vi "MagnetometerStateMachineV1.vi"() -> ()   [LabVIEW 2014]
uses:
  <vilib>/MakerHub/LINX/Private/Local IO/LinxI2cWrite.vi
  <vilib>/MakerHub/LINX/Public/Utilities/Check Channel.vi
  <vilib>/MakerHub/LINX/Public/Utilities/Open Serial.vi
  <vilib>/MakerHub/LINX/Private/Utilties/Generate Error.vi
  <instrlib>/Stanford Research 830/Public/Data/Read (All Parameters).vi
  <vilib>/MakerHub/LINX/LMH-LINX.lvlib
  <instrlib>/Stanford Research 830/Stanford Research 830.lvlib
panel:
  out "SRS-T":dbl
  out "SRS-R":dbl
  out "SRS-Y":dbl
  out "Parameter Values":T1
  out "XY Graph":T2(graph)
  out "SRS-X":dbl
  in  "Time Constant (8: 100ms)":u16(ring)=8 items=["10 us", "30 us", "100 us", "300 us", "1 ms", "3 ms", "10 ms", "30 ms", "100 ms", "300 ms", "1 s", "3 s", "10 s", "30 s", "100 s", "300 s", "1 ks", "3 ks", "10 ks", "30 ks"]
  in  "Internal Reference Frequency (1000 Hz)":dbl=1000.0
  in  "Sine Output Amplitude (1 V)":dbl=1.0
  in  "Sensitivity (26: 1 V/uA)":i16(ring)=26 items=["Auto Gain"=-1, "2 nV/fA"=0, "5 nV/fA"=1, "10 nV/fA"=2, "20 nV/fA"=3, "50 nV/fA"=4, "100 nV/fA"=5, "200 nV/fA"=6, "500 nV/fA"=7, "1 uV/pA"=8, "2 uV/pA"=9, "5 uV/pA"=10, "10 uV/pA"=11, "20 uV/pA"=12, "50 uV/pA"=13, "100 uV/pA"=14, "200 uV/pA"=15, "500 uV/pA"=16, "1 mV/nA"=17, "2 mV/nA"=18, "5 mV/nA"=19, "10 mV/nA"=20, "20 mV/nA"=21, "50 mV/nA"=22, "100 mV/nA"=23, "200 mV/nA"=24, "500 mV/mA"=25, "1 V/uA"=26]
  in  "Dynamic Reserve (2: Low Noise)":i16(ring)=2 items=["High Reserve"=0, "Normal"=1, "Low Noise"=2, "Auto Reserve"=-1]
  in  "Reference Source (1: Internal)":u16(ring)=1 items=["External", "Internal"]
  in  "Input Coupling (0: AC)":u16(ring) items=["AC", "DC"]
  in  "Input Connection (0: Single-Ended Voltage)":u16(ring) items=["Single-Ended Voltage", "Differential Voltage", "1 MOhm Current Gain", "100 MOhm Current Gain"]
  in  "Current DAC Value":dbl
  in  "Max H Field (Oe)":sgl min=0 max=900 step=0.1
  in  "DAC Zeroing Voltage":dbl=2.5 min=0.0 max=5.0 step=0.001 format="%#_6f"
  out "Magnetic Field (Oe)":dbl
  in  "Choices":T3(ring)
  in  "End It All!":bool
  out "Error Out":errorcluster={"status"=FALSE, "code"=1073676294, "source"="VISA Read in LVH-LINX.lvlib:Device.lvlib:Serial Read.vi->LVH-LINX.lvlib:Device.lvlib:Wait For Packet.vi->LVH-LINX.lvlib:Device.lvlib:Send Command.vi->LVH-LINX.lvlib:Device.lvlib:Get DIO Channels.vi->LVH-LINX.lvlib:Device.lvlib:Load Device Config.vi->LVH-LINX.lvlib:Device.lvlib:Initialize Device.vi->LVH-LINX.lvlib:Initialize.vi->Untitled 2"}
  out "Device Name":string
  in  "Arduino Port":refnum<visa-resource-name>="N/A"
  # "Enter the voltage to get\nthe magnetic field to be zero."
  # "Input Signal"
  # "Reference"
  # "Sensitivity and Reserve"
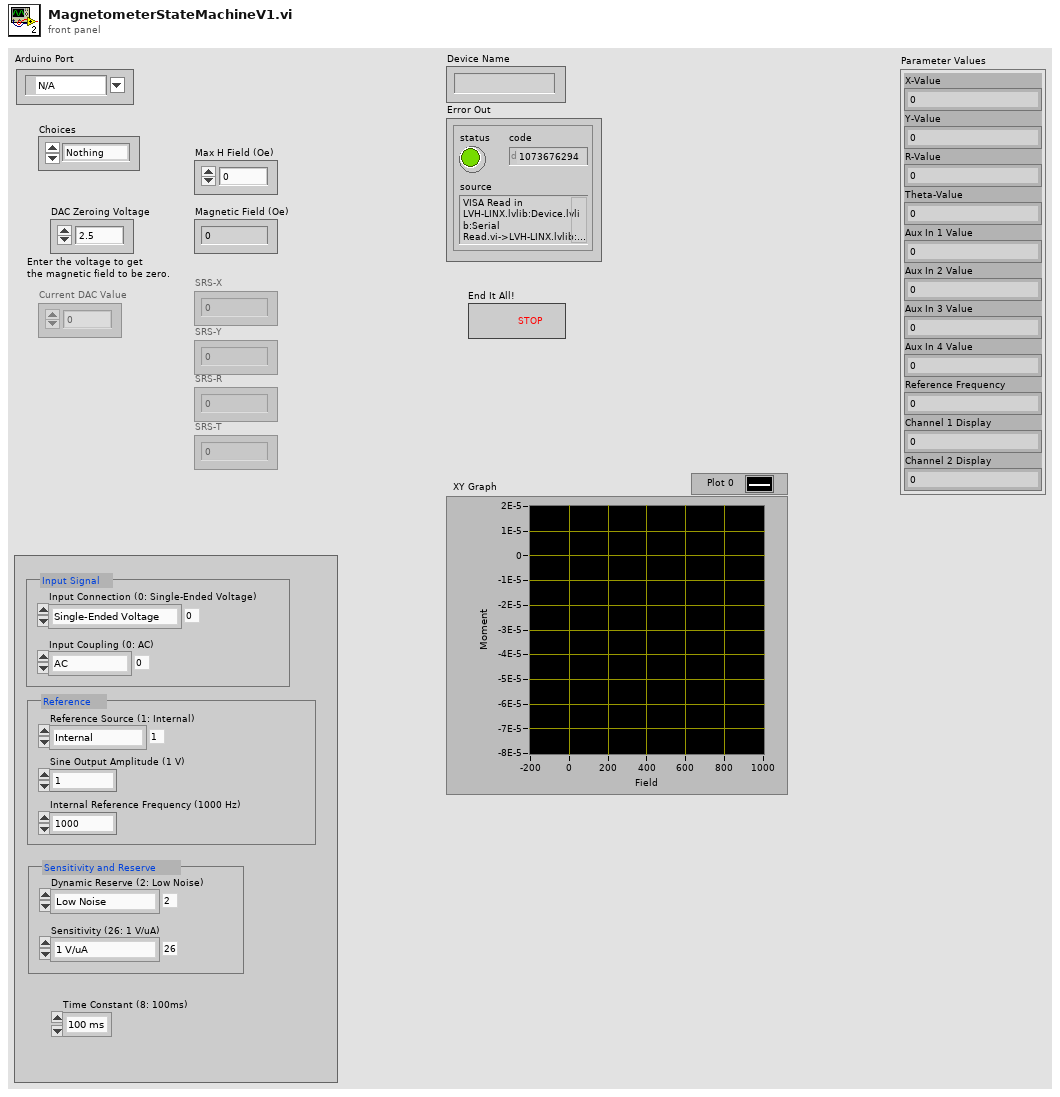
[diagram p1: front panel]
types:
  T1 = cluster{"X-Value":dbl, "Y-Value":dbl, "R-Value":dbl, "Theta-Value":dbl, "Aux In 1 Value":dbl, "Aux In 2 Value":dbl, "Aux In 3 Value":dbl, "Aux In 4 Value":dbl, "Reference Frequency":dbl, "Channel 1 Display":dbl, "Channel 2 Display":dbl}
  T2 = cluster{"Magnetic Field (Oe)":dbl, "Moment":dbl}[]
  T3 = enum16{"Nothing", "Hysteresis", "MvsT", "SetTemperature", "ZeroHField"}
  T4 = typedef "LMH-LINX.lvlib/LINX Ref.ctl" = cluster{"IO":T5, "Interface":T6, "LINX Device Config":T7}
  T5 = typedef "LMH-LINX.lvlib/Platform.ctl" = enum16{"Remote", "Local"}
  T6 = typedef "LMH-LINX.lvlib/Interface.ctl" = enum16{"Serial", "TCP"}
  T7 = typedef "LMH-LINX.lvlib/Device.lvlib/LINX Device Config.ctl" = cluster{"Interface":T6, "COM Port":refnum<visa-resource-name>, "TCP Configuration":T8, "Device Family":u8, "Device ID":u8, "Device Name":string, "TCP Ref":refnum<k5>, "Channels":T9}
  T8 = typedef "LMH-LINX.lvlib/Device.lvlib/TCP Config.ctl" = cluster{"IP Address":string, "Port":u16}
  T9 = typedef "LMH-LINX.lvlib/Channels.ctl" = cluster{"DI":u8[], "DO":u8[], "AI":u8[], "AO":u8[], "PWM":u8[], "QE":u8[], "UART":u8[], "I2C 2":u8[], "SPI":u8[], "CAN":u8[], "Servo":u8[], "AI Ref (V)":dbl, "AI Resolution (Bits)":u8, "AO Ref (V)":dbl, "AO Resolution (Bits)":u8}
  T10 = cluster{"Magnetic Field (Oe)":dbl, "SRS-X":dbl}[]
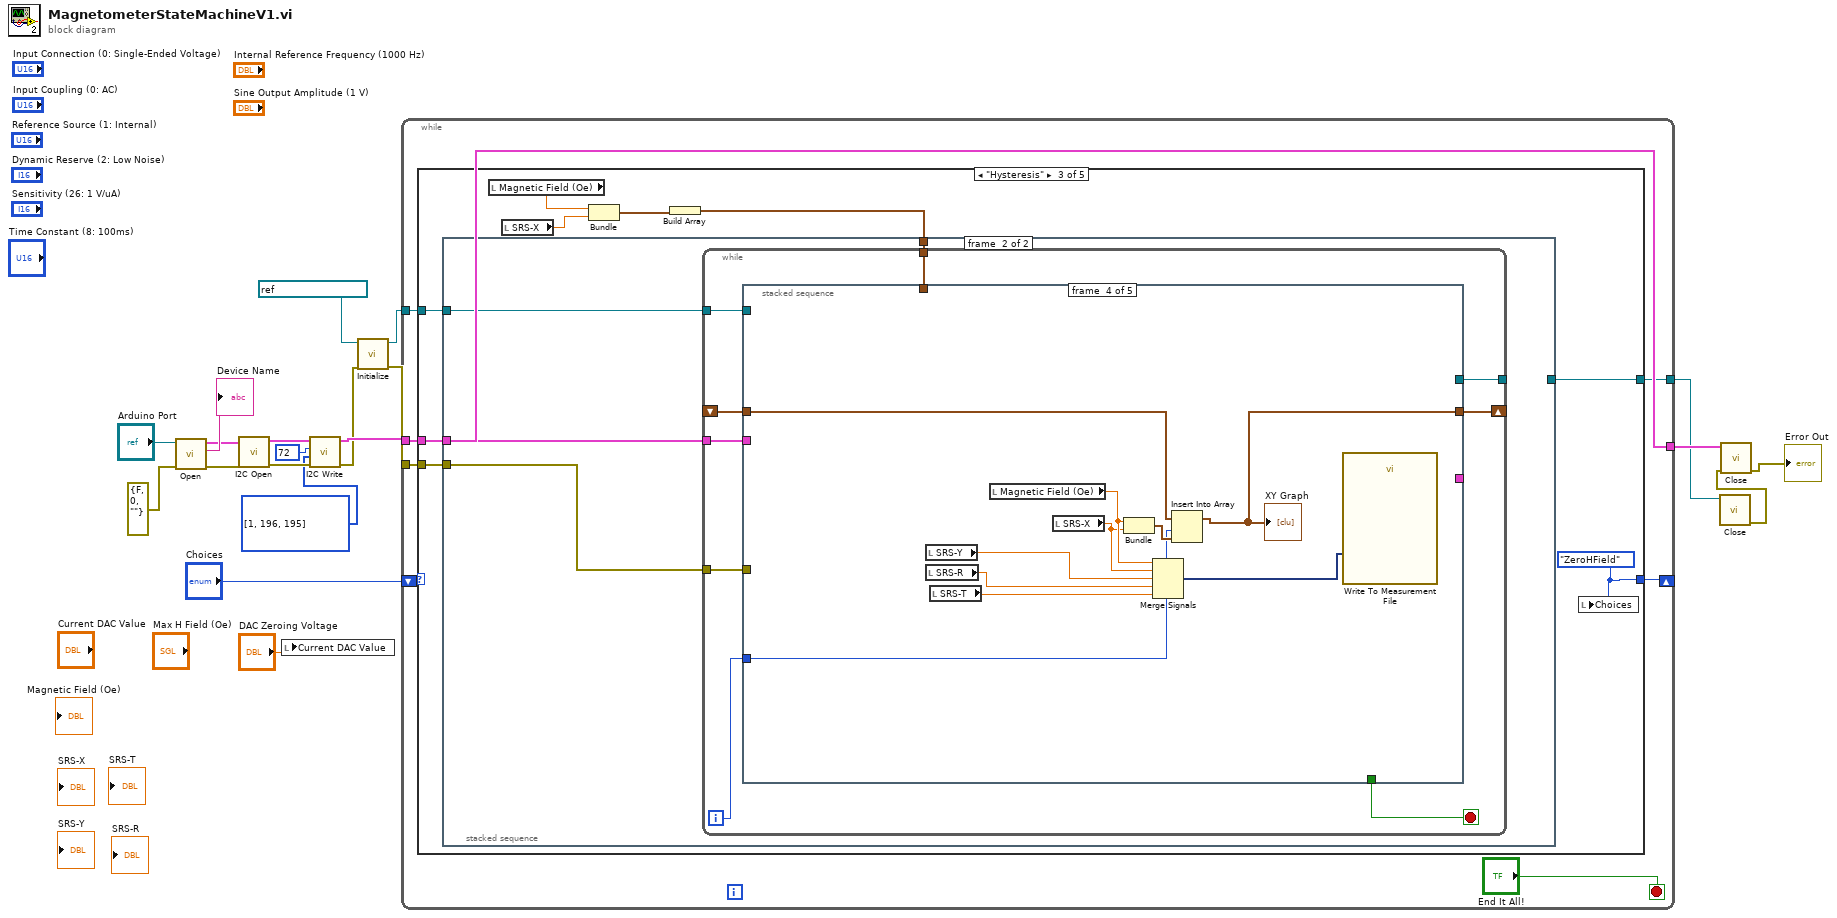
[diagram p0: block diagram]
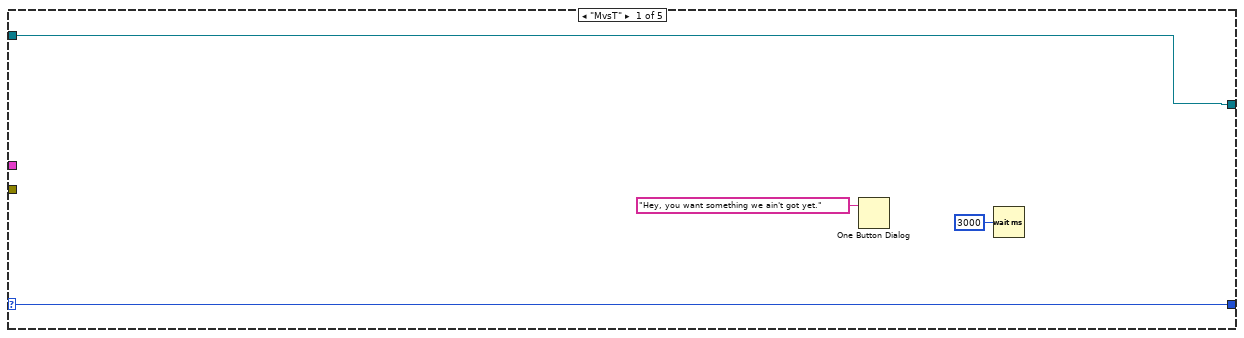
[diagram p2: hidden frame]
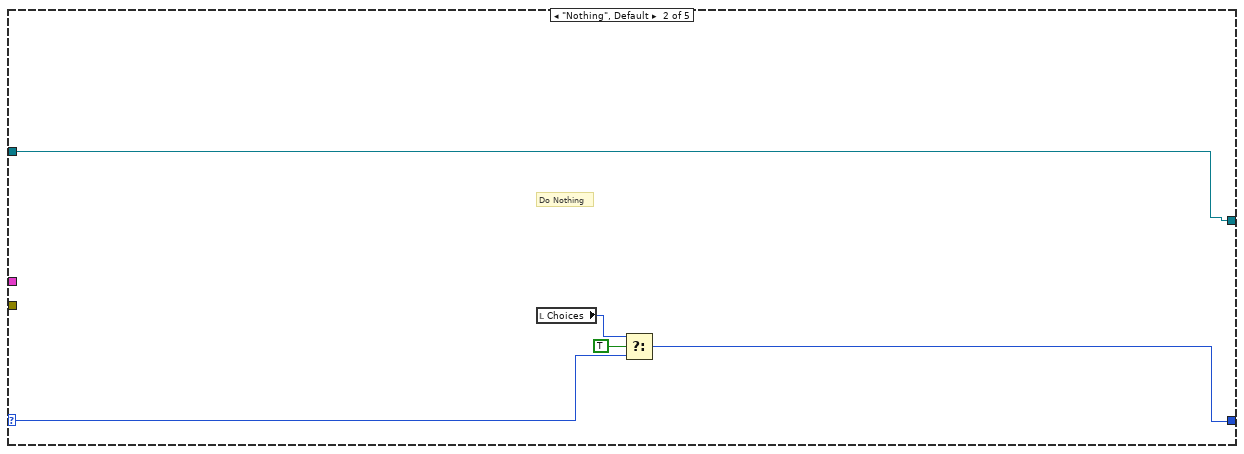
[diagram p3: hidden frame]
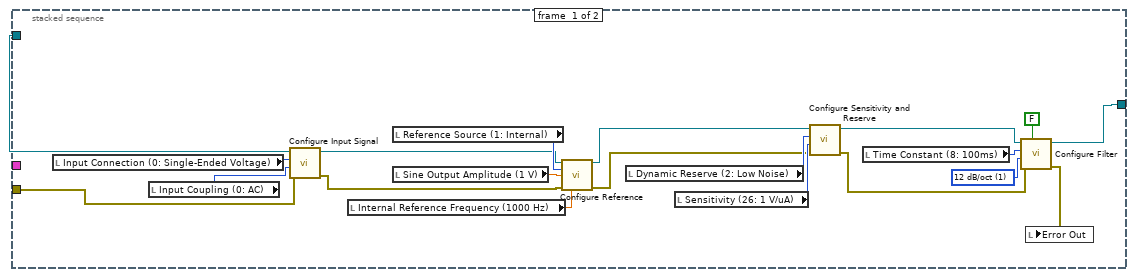
[diagram p4: hidden frame]
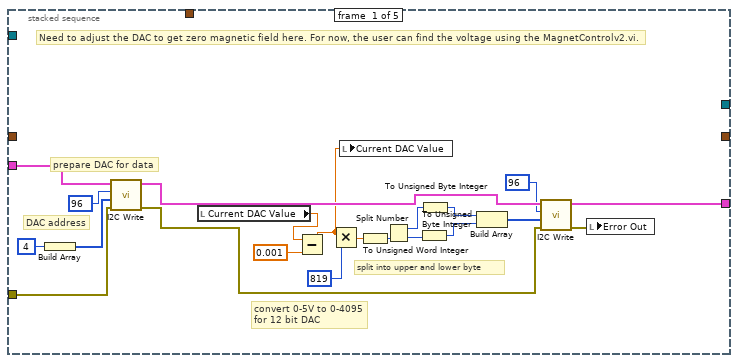
[diagram p5: hidden frame]
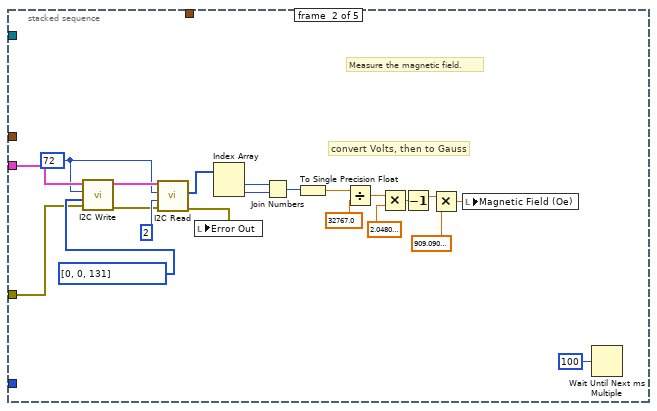
[diagram p6: hidden frame]
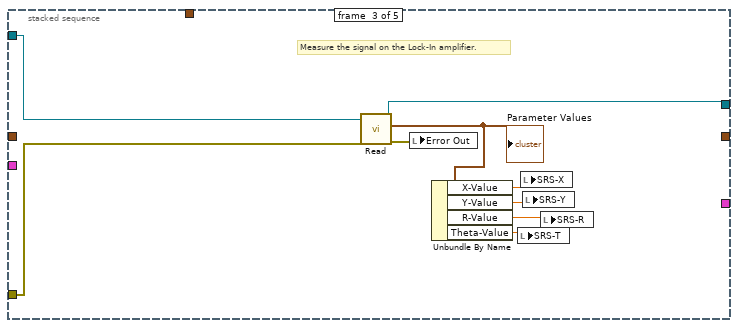
[diagram p7: hidden frame]
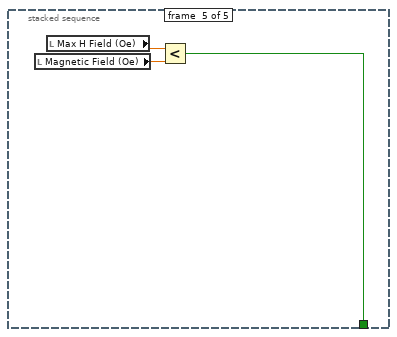
[diagram p8: hidden frame]
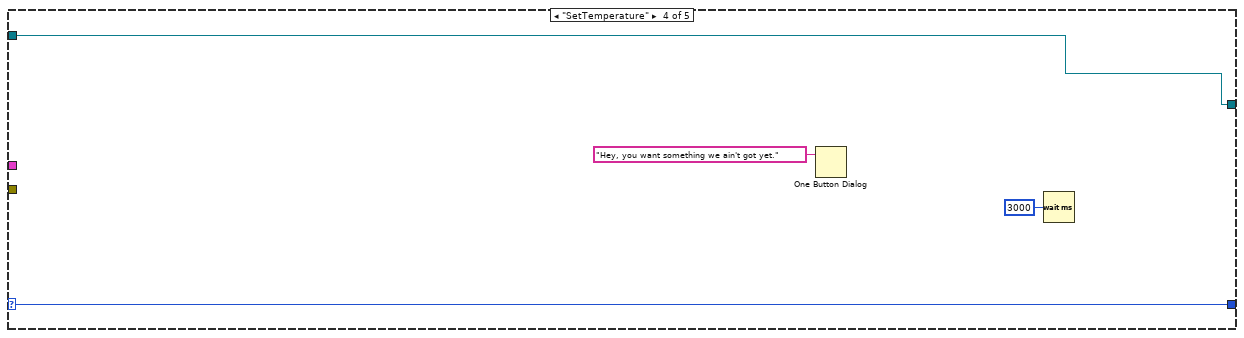
[diagram p9: hidden frame]
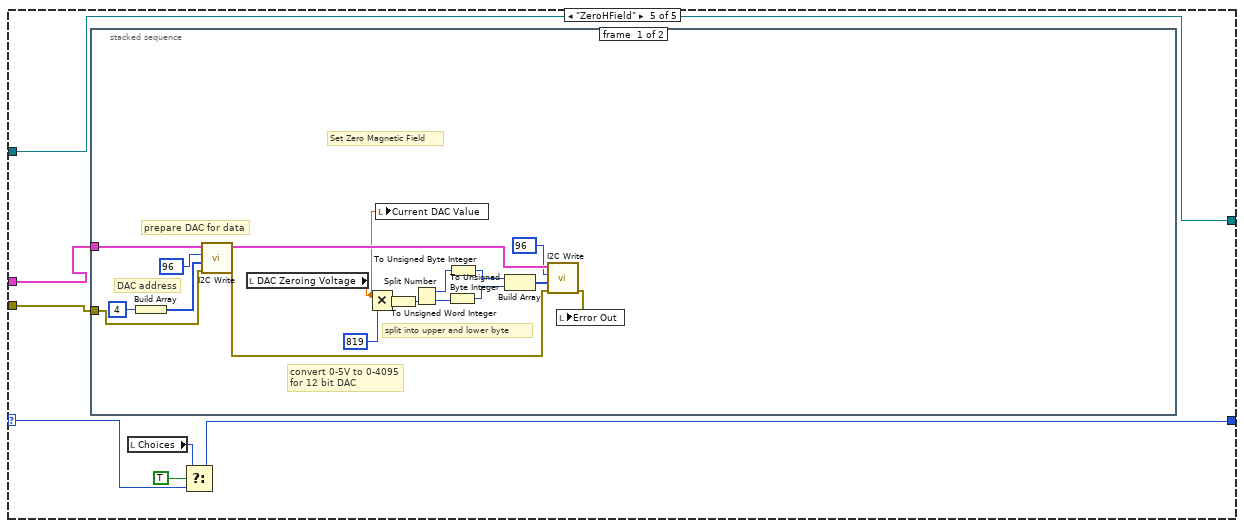
[diagram p10: hidden frame]
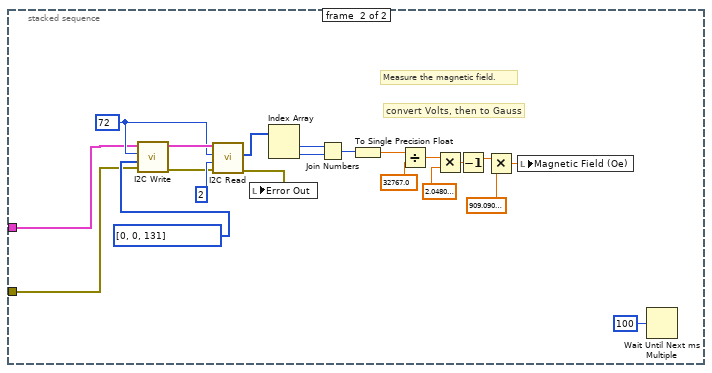
[diagram p11: hidden frame]
diagram:
  n1 = call-poly <vilib>:"Open.vi"("Error In"=errorcluster {"status"=FALSE, "code"=0, "source"=""}, "Serial Port"="Arduino Port") -> ("Error Out"=w15:errorcluster, "Device Name"=→"Device Name":string, "LINX Resource"=w16:T4)  [unwired: 7 in]
  n2 = call <vilib>:"I2C Open.vi"("Error In"=w15, "LINX Resource"=w16) -> ("Error Out"=w10:errorcluster, "LINX Resource"=w11:T4)  [unwired: 8 in]
  n3 = local write "Current DAC Value"("DAC Zeroing Voltage") -> ()
  n4 = call <vilib>:"I2C Write.vi"("Error In"=w10, "Data"=u8[] [1, 196, 195], "I2C Slave Address (0)"=u8 72, "LINX Resource"=w11) -> ("Error Out"=w5:errorcluster, "LINX Resource"=w12:T4)  [unwired: 6 in]
  n5 = call <instrlib>:"Initialize.vi"("error in (no error)"=w5, "VISA resource name"=refnum<visa-resource-name> "GPIB0::8::INSTR") -> ("error out"=w4:errorcluster, "VISA resource name out"=w3:refnum<visa-resource-name>)  [unwired: 8 in]
  n6 = while {
    shift-right: [w24] -> _
    shift-left: "Choices" -> [w26]
    tunnel: w12 -> [w23]
    tunnel: w4 -> [w25]
    tunnel: [w23] -> w13
    tunnel: w3 -> [w22]
    tunnel: [w21] -> w2
    stop <- "End It All!" stop-if-true
    n7 = case shown="\"Hysteresis\"" w26 {
      selector: w26 -> [w30 w36 _ w145 w153]
      tunnel: w25 -> [_ _ w39 _ w152]
      tunnel: w23 -> [_ _ w45 _ w151]
      tunnel: [w30 w34 w44 w145 w150] -> w24
      tunnel: w22 -> [w28 w32 w41 w143 w147]
      tunnel: [w28 w32 w40 w143 w147] -> w21
      frame "MvsT" {
        n8 = One Button Dialog(message="Hey, you want something we ain't got yet.") -> ()  [unwired: 1 in, 1 out]
        n9 = Wait (ms)(milliseconds to wait=u32 3000) -> ()  [unwired: 1 out]
      }
      frame "Nothing", Default {
        # "Do Nothing"
        n10 = local read "Choices"() -> (w35:T3)
        n11 = Select(t=w35, s=TRUE, f=w36) -> (s? t:f=w34:T3)
      }
      frame "Hysteresis" {
        w44 = T3."ZeroHField"
        n12 = local read "Magnetic Field (Oe)"() -> (w38:dbl)
        n13 = local read "SRS-X"() -> (w37:dbl)
        n14 = Bundle("Magnetic Field (Oe)"=w38, "SRS-X"=w37) -> (w42:cluster{"Magnetic Field (Oe)":dbl, "SRS-X":dbl})  [unwired: 1 in]
        n15 = Build Array(w42) -> (w43:T10)
        n16 = stacked-sequence {
          tunnel: w45 -> [_ w69]
          tunnel: w43 -> [_ w68]
          tunnel: w41 -> [w56 w67]
          tunnel: [w52 _] -> w40
          tunnel: w39 -> [w51 w66]
          frame #0 {
            w58 = u16 1 items=["6 dB/oct", "12 dB/oct", "18 db/oct", "24 dB/oct"] ("Low Pass Filter Slope (1: 12dB/oct)")
            n17 = local read "Input Connection (0: Single-Ended Voltage)"() -> (w65:u16)
            n18 = local read "Input Coupling (0: AC)"() -> (w64:u16)
            n19 = call <instrlib>:"Configure Input Signal.vi"("error in (no error)"=w51, "Input Coupling (0: AC)"=w64, "Input Connection (0: Single-Ended Voltage)"=w65, "VISA resource name"=w56) -> ("error out"=w50:errorcluster, "VISA resource name out"=w55:refnum<visa-resource-name>)  [unwired: 6 in]
            n20 = local read "Internal Reference Frequency (1000 Hz)"() -> (w61:dbl)
            n21 = local read "Reference Source (1: Internal)"() -> (w62:u16)
            n22 = local read "Sine Output Amplitude (1 V)"() -> (w63:dbl)
            n23 = call <instrlib>:"Configure Reference.vi"("VISA resource name"=w55, "Reference Source (1: Internal)"=w62, "Sine Output Amplitude (1 V)"=w63, "error in (no error)"=w50, "Internal Reference Frequency (1000 Hz)"=w61) -> ("VISA resource name out"=w54:refnum<visa-resource-name>, "error out"=w49:errorcluster)  [unwired: 9 in]
            n24 = local read "Dynamic Reserve (2: Low Noise)"() -> (w59:i16)
            n25 = local read "Sensitivity (26: 1 V/uA)"() -> (w60:i16)
            n26 = call <instrlib>:"Configure Sensitivity and Reserve.vi"("error in (no error)"=w49, "Sensitivity (-1: Auto gain)"=w60, "Dynamic Reserve (-1: Auto Reserve)"=w59, "VISA resource name"=w54) -> ("error out"=w48:errorcluster, "VISA resource name out"=w53:refnum<visa-resource-name>)  [unwired: 6 in]
            n27 = local read "Time Constant (8: 100ms)"() -> (w57:u16)
            n28 = call <instrlib>:"Configure Filter.vi"("Enable Sync Filter (F: Disable)"=FALSE, "error in (no error)"=w48, "Low Pass Filter Slope (1: 12dB/oct)"=w58, "Time Constant (8: 100ms)"=w57, "VISA resource name"=w53) -> ("error out"=w46:errorcluster, "VISA resource name out"=w52:refnum<visa-resource-name>)  [unwired: 5 in]
            n29 = local write "Error Out"(w46) -> ()
          }
          frame #1 {
            n30 = while {
              tunnel: w66 -> [w77]
              tunnel: w69 -> [w78]
              tunnel: w67 -> [w75]
              tunnel: w68 -> [w73]
              tunnel: [w72] -> _
              shift-right: [w71] -> _
              shift-left: _ -> [w70]
              i -> [w74]
              stop <- w76 stop-if-true
              n31 = stacked-sequence {
                tunnel: [w99 _ _ _ _] -> _
                tunnel: w78 -> [w98 w104 _ _ _]
                tunnel: w77 -> [w92 w103 w127 _ _]
                tunnel: [_ _ _ _ w140] -> w76
                tunnel: w75 -> [_ _ w128 _ _]
                tunnel: w74 -> [_ _ _ w138 _]
                tunnel: w73 -> [_ _ _ _ _]
                tunnel: [_ _ w126 _ _] -> w72
                tunnel: [_ _ _ w137 _] -> w71
                tunnel: w70 -> [_ _ _ w136 _]
                frame #0 {
                  # "convert 0-5V to 0-4095\nfor 12 bit DAC"
                  # "split into upper and lower byte"
                  # "Need to adjust the DAC to get zero magnetic field here. For now, the user can find the voltage using the MagnetControlv2.vi."
                  # "DAC address"
                  # "prepare DAC for data"
                  n32 = Build Array(u8 4) -> (w93:u8[])
                  n33 = call <vilib>:"I2C Write.vi"("Error In"=w92, "Data"=w93, "I2C Slave Address (0)"=u8 96, "LINX Resource"=w98) -> ("Error Out"=w96:errorcluster, "LINX Resource"=w95:T4)  [unwired: 6 in]
                  n34 = local read "Current DAC Value"() -> (w81:dbl)
                  n35 = Subtract(x=w81, y=0.001) -> (x-y=w79:dbl)
                  n36 = Multiply(x=w79, y=u32 819) -> (x*y=w83:dbl)
                  n37 = local write "Current DAC Value"(w79) -> ()
                  n38 = To Unsigned Word Integer(number=w83) -> (unsigned 16bit integer=w85:u16)
                  n39 = Split Number(x=w85) -> (hi(x)=w86:u8, lo(x)=w90:u8)
                  n40 = To Unsigned Byte Integer(number=w90) -> (unsigned 8bit integer=w88:u8)
                  n41 = To Unsigned Byte Integer(number=w86) -> (unsigned 8bit integer=w89:u8)
                  n42 = Build Array(w89, w88) -> (w87:u8[])
                  n43 = call <vilib>:"I2C Write.vi"("Error In"=w96, "Data"=w87, "I2C Slave Address (0)"=u8 96, "LINX Resource"=w95) -> ("Error Out"=w82:errorcluster, "LINX Resource"=w99:T4)  [unwired: 6 in]
                  n44 = local write "Error Out"(w82) -> ()
                }
                frame #1 {
                  w102 = u8 72 ("I2C Slave Address (0)")
                  # "Measure the magnetic field."
                  # "convert Volts, then to Gauss"
                  n45 = call <vilib>:"I2C Write.vi"("Error In"=w103, "Data"=u8[] [0, 0, 131], "I2C Slave Address (0)"=w102, "LINX Resource"=w104) -> ("Error Out"=w116:errorcluster, "LINX Resource"=w117:T4)  [unwired: 6 in]
                  n46 = call <vilib>:"I2C Read.vi"("Error In"=w116, "Bytes To Read"=u8 2, "I2C Slave Address (0)"=w102, "LINX Resource"=w117) -> ("Error Out"=w105:errorcluster, "Data"=w119:u8[])  [unwired: 5 in, 1 out]
                  n47 = local write "Error Out"(w105) -> ()
                  n48 = Index Array(array=w119) -> (element #1=w113:u8, element #2=w112:u8)  [unwired: 2 in]
                  n49 = Join Numbers(hi=w113, lo=w112) -> ((hi.lo)=w115:u16)
                  n50 = To Single Precision Float(number=w115) -> (single precision float=w108:sgl)
                  n51 = Divide(x=w108, y=sgl 32767.0) -> (x/y=w111:sgl)
                  n52 = Multiply(x=w111, y=sgl 2.048) -> (x*y=w110:sgl)
                  n53 = Decrement(x=w110) -> (x-1=w106:sgl)
                  n54 = Multiply(x=w106, y=sgl 909.09) -> (x*y=w101:sgl)
                  n55 = local write "Magnetic Field (Oe)"(w101) -> ()
                  n56 = Wait Until Next ms Multiple(millisecond multiple=u32 100) -> ()  [unwired: 1 out]
                }
                frame #2 {
                  # "Measure the signal on the Lock-In amplifier."
                  n57 = call-poly <instrlib>:"Read.vi"("error in (no error)"=w127, "VISA resource name"=w128) -> ("error out"=w129:errorcluster, "Parameter Values"=w125:T1, "VISA resource name out"=w126:refnum<visa-resource-name>)  [unwired: 7 in]
                  "Parameter Values" <- w125
                  n58 = local write "Error Out"(w129) -> ()
                  n59 = Unbundle By Name(w125) -> ("X-Value"=w123:dbl, "Y-Value"=w121:dbl, "R-Value"=w124:dbl, "Theta-Value"=w122:dbl)
                  n60 = local write "SRS-T"(w122) -> ()
                  n61 = local write "SRS-X"(w123) -> ()
                  n62 = local write "SRS-Y"(w121) -> ()
                  n63 = local write "SRS-R"(w124) -> ()
                }
                frame #3 {
                  n64 = local read "SRS-Y"() -> (w132:dbl)
                  n65 = local read "SRS-R"() -> (w131:dbl)
                  n66 = local read "SRS-T"() -> (w130:dbl)
                  n67 = local read "Magnetic Field (Oe)"() -> (w135:dbl)
                  n68 = local read "SRS-X"() -> (w133:dbl)
                  n69 = Bundle("Magnetic Field (Oe)"=w135, "SRS-X"=w133) -> (w139:cluster{"Magnetic Field (Oe)":dbl, "SRS-X":dbl})  [unwired: 1 in]
                  n70 = Merge Signals(w135, w133, w132, w131, w130) -> (w134:dynamicdata)
                  n71 = Insert Into Array(array=w136, index=w138, new element=w139) -> (w137:T10)
                  "XY Graph" <- w137
                  n72 = call "Write To Measurement File"("Signals"=w134) -> ()  [unwired: 16 in, 3 out]
                }
                frame #4 {
                  n73 = local read "Magnetic Field (Oe)"() -> (w141:dbl)
                  n74 = local read "Max H Field (Oe)"() -> (w142:sgl)
                  n75 = Less?(x=w142, y=w141) -> (x < y?=w140:bool)
                }
              }
            }
          }
        }
        n76 = local write "Choices"(w44) -> ()
      }
      frame "SetTemperature" {
        n77 = One Button Dialog(message="Hey, you want something we ain't got yet.") -> ()  [unwired: 1 in, 1 out]
        n78 = Wait (ms)(milliseconds to wait=u32 3000) -> ()  [unwired: 1 out]
      }
      frame "ZeroHField" {
        n79 = stacked-sequence {
          tunnel: w152 -> [w157 w172]
          tunnel: w151 -> [w155 w173]
          frame #0 {
            # "convert 0-5V to 0-4095\nfor 12 bit DAC"
            # "split into upper and lower byte"
            # "DAC address"
            # "prepare DAC for data"
            # "Set Zero Magnetic Field"
            n80 = Build Array(u8 4) -> (w167:u8[])
            n81 = call <vilib>:"I2C Write.vi"("Error In"=w157, "Data"=w167, "I2C Slave Address (0)"=u8 96, "LINX Resource"=w155) -> ("Error Out"=w170:errorcluster, "LINX Resource"=w169:T4)  [unwired: 6 in]
            n82 = local read "DAC Zeroing Voltage"() -> (w156:dbl)
            n83 = Multiply(x=w156, y=u32 819) -> (x*y=w158:dbl)
            n84 = local write "Current DAC Value"(w156) -> ()
            n85 = To Unsigned Word Integer(number=w158) -> (unsigned 16bit integer=w160:u16)
            n86 = Split Number(x=w160) -> (hi(x)=w161:u8, lo(x)=w165:u8)
            n87 = To Unsigned Byte Integer(number=w165) -> (unsigned 8bit integer=w163:u8)
            n88 = To Unsigned Byte Integer(number=w161) -> (unsigned 8bit integer=w164:u8)
            n89 = Build Array(w164, w163) -> (w162:u8[])
            n90 = call <vilib>:"I2C Write.vi"("Error In"=w170, "Data"=w162, "I2C Slave Address (0)"=u8 96, "LINX Resource"=w169) -> ("Error Out"=w154:errorcluster)  [unwired: 6 in, 1 out]
            n91 = local write "Error Out"(w154) -> ()
          }
          frame #1 {
            w176 = u8 72 ("I2C Slave Address (0)")
            # "Measure the magnetic field."
            # "convert Volts, then to Gauss"
            n92 = call <vilib>:"I2C Write.vi"("Error In"=w172, "Data"=u8[] [0, 0, 131], "I2C Slave Address (0)"=w176, "LINX Resource"=w173) -> ("Error Out"=w188:errorcluster, "LINX Resource"=w189:T4)  [unwired: 6 in]
            n93 = call <vilib>:"I2C Read.vi"("Error In"=w188, "Bytes To Read"=u8 2, "I2C Slave Address (0)"=w176, "LINX Resource"=w189) -> ("Error Out"=w177:errorcluster, "Data"=w191:u8[])  [unwired: 5 in, 1 out]
            n94 = local write "Error Out"(w177) -> ()
            n95 = Index Array(array=w191) -> (element #1=w185:u8, element #2=w184:u8)  [unwired: 2 in]
            n96 = Join Numbers(hi=w185, lo=w184) -> ((hi.lo)=w187:u16)
            n97 = To Single Precision Float(number=w187) -> (single precision float=w180:sgl)
            n98 = Divide(x=w180, y=sgl 32767.0) -> (x/y=w183:sgl)
            n99 = Multiply(x=w183, y=sgl 2.048) -> (x*y=w182:sgl)
            n100 = Decrement(x=w182) -> (x-1=w178:sgl)
            n101 = Multiply(x=w178, y=sgl 909.09) -> (x*y=w175:sgl)
            n102 = local write "Magnetic Field (Oe)"(w175) -> ()
            n103 = Wait Until Next ms Multiple(millisecond multiple=u32 100) -> ()  [unwired: 1 out]
          }
        }
        n104 = local read "Choices"() -> (w149:T3)
        n105 = Select(t=w149, s=TRUE, f=w153) -> (s? t:f=w150:T3)
      }
    }
  }
  n106 = call <vilib>:"Close.vi"("VISA resource name"=w2) -> ("error out"=w1:errorcluster)  [unwired: 10 in]
  n107 = call <vilib>:"Close.vi"("Error In"=w1, "LINX Resource"=w13) -> ("Error Out"=→"Error Out":errorcluster)  [unwired: 9 in]
